vi "Host - Get HW Config.vi"(8 "error in (no error)":errorcluster, 11 "serverName":string="10.0.18.244") -> (0 "error out":errorcluster, 3 "HW Config":T1)   [LabVIEW 2019, in "SEECD System Explorer.lvlib"]
uses:
  SEECD System Explorer.lvlib
  Type Defs/Host - HW Config.ctl
  Type Defs/Host - Local Chassis.ctl
  Type Defs/Host - Module.ctl
  Type Defs/IOV Container Contents.ctl
  Type Defs/Host - Master.ctl
  Type Defs/Host - Slave.ctl
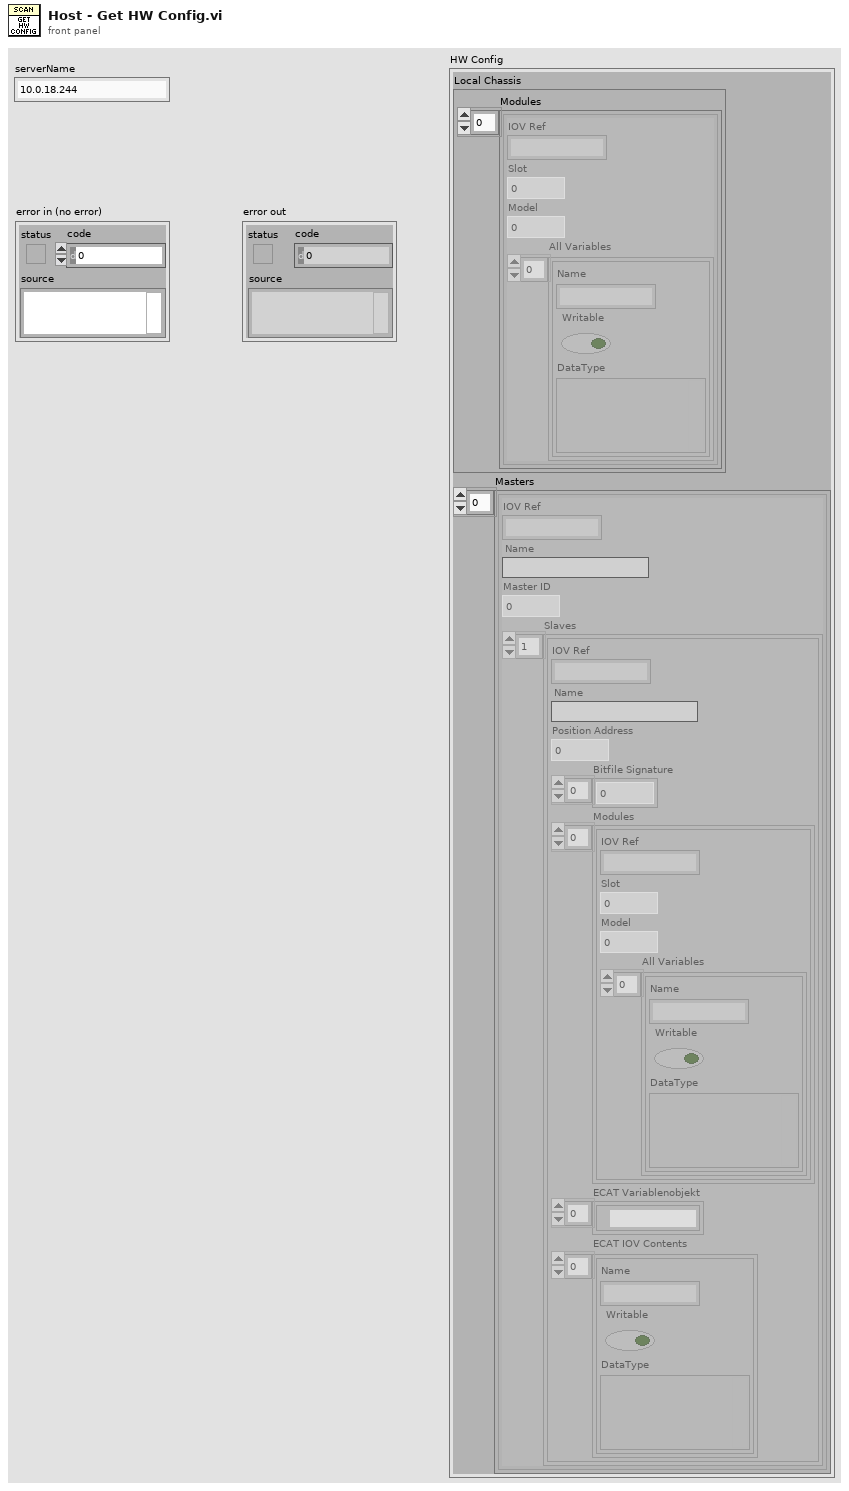
[diagram p1: front panel]
types:
  T1 = typedef "SEECD System Explorer.lvlib/Host - HW Config.ctl" = cluster{"Local Chassis":T2, "Masters":T5[]}
  T2 = typedef "SEECD System Explorer.lvlib/Host - Local Chassis.ctl" = cluster{"Modules":T3[]}
  T3 = typedef "SEECD System Explorer.lvlib/Host - Module.ctl" = cluster{"IOV Ref":string, "Slot":u32, "Model":u32, "All Variables":T4[]}
  T4 = typedef "SEECD System Explorer.lvlib/IOV Container Contents.ctl" = cluster{"Name":string, "Writable":bool, "DataType":variant}
  T5 = typedef "SEECD System Explorer.lvlib/Host - Master.ctl" = cluster{"IOV Ref":string, "Name":string, "Master ID":u32, "Slaves":T6[]}
  T6 = typedef "SEECD System Explorer.lvlib/Host - Slave.ctl" = cluster{"IOV Ref":string, "Name":string, "Position Address":u16, "Bitfile Signature":u8[], "Modules":T3[], "ECAT Variablenobjekt":refnum<k21>[], "ECAT IOV Contents":T4[]}
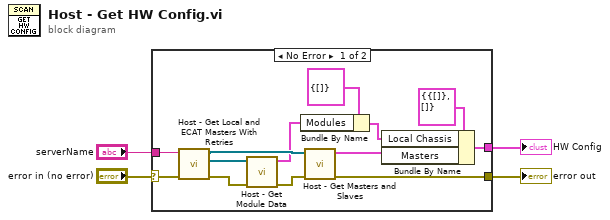
[diagram p0: block diagram]
diagram:
  n1 = case shown="No Error" "error in (no error)" {
    selector: "error in (no error)" -> [w15 w18]
    tunnel: "serverName" -> [w17 _]
    tunnel: [w14 w18] -> w3
    tunnel: [w10 _] -> w1
    frame No Error {
      n2 = call "Host - Get Local and ECAT Masters With Retries.vi"("error in (no error)"=w15, "serverName"=w17) -> ("error out"=w5:errorcluster, "All Local Mods"=w13:refnum<k21>[], "All ECAT Masters"=w16:refnum<k21>[])  [unwired: 7 in]
      n3 = call "Host - Get Module Data.vi"("error in (no error)"=w5, "Mod IOVs"=w13) -> ("error out"=w9:errorcluster, "Modules"=w7:T3[])  [unwired: 8 in]
      n4 = Bundle By Name(cluster=T2 {"Modules"=[]} ("Local Chassis"), "Modules"=w7) -> (w6:T2)
      n5 = call "Host - Get Masters and Slaves.vi"("error in (no error)"=w9, "All ECAT Masters"=w16) -> ("error out"=w14:errorcluster, "Array"=w11:T5[])  [unwired: 8 in]
      n6 = Bundle By Name(cluster=T1 {"Local Chassis"={"Modules"=[]}, "Masters"=[]} ("HW Config"), "Local Chassis"=w6, "Masters"=w11) -> (w10:T1)
    }
    frame Error {
    }
  }
  "error out" <- w3
  "HW Config" <- w1
